vi "Format Version Number.vi"(8 "error in (no error)":errorcluster, 10 "Number of Digits (4)":i32=4, 11 "Version In":string) -> (0 "error out":errorcluster, 3 "Version Out":string)   [LabVIEW 2014, in "SLL Utilities.lvlib"]
doc: "Formats the version number to be in the required number of digits. \n\nEg: If version input is 1.0 and the number of digits is 4, then version out will be 1.0.0.0\n\nIf the number of digits is specified as -1 or 0, it will ignore the operation."
uses:
  SLL Utilities.lvlib
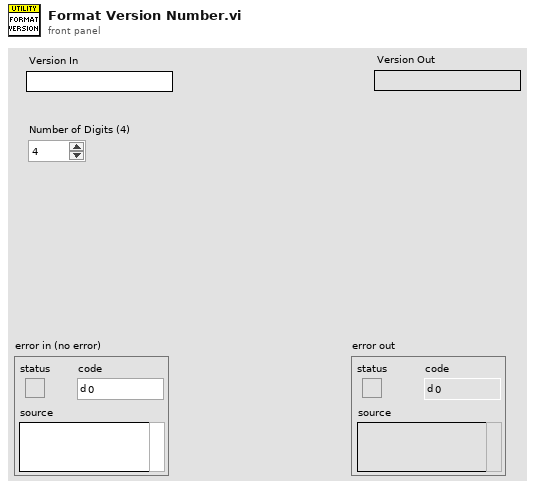
[diagram p1: front panel]
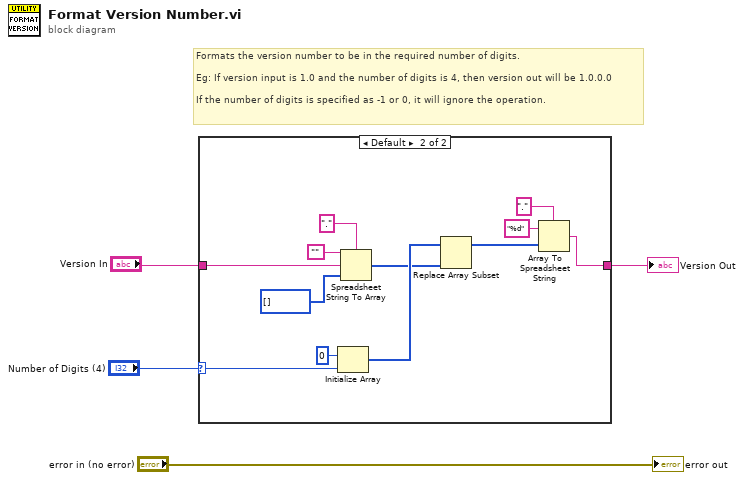
[diagram p0: block diagram]
diagram:
  # "Formats the version number to be in the required number of digits. \n\nEg: If version input is 1.0 and the number of digits is 4, then version out will be 1.0.0.0\n\nIf the number of digits is specified as -1 or 0, it will ignore the operation."
  n1 = case shown="Default" "Number of Digits (4)" {
    selector: "Number of Digits (4)" -> [_ w15]
    tunnel: [w5 w17] -> w3
    tunnel: "Version In" -> [w5 w16]
    frame -1, 0 {
      # "Retain the input version number"
    }
    frame Default {
      n2 = Initialize Array(u32 0 ("element"), w15) -> (w10:u32[])
      n3 = Spreadsheet String To Array(delimiter (Tab)=".", format string="", spreadsheet string=w16, array type (2D Dbl)=u32[] []) -> (array=w9:u32[])
      n4 = Replace Array Subset(array=w10, new element=w9) -> (w8:u32[])  [unwired: 1 in]
      n5 = Array To Spreadsheet String(delimiter (Tab)=".", array=w8, 3:"%d" ("format string")) -> (spreadsheet string=w17:string)
    }
  }
  "Version Out" <- w3
  "error out" <- "error in (no error)"
